vi "NiFpgaDEN_SimulationStrings.vi"() -> ()   [LabVIEW 2017]
panel:
  in  "DEN Simulation VI Tag":string="niFpgaSimulateUnderDEN"
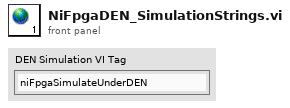
[diagram p1: front panel]
diagram:
